vi "load control code.vi"(2 "Switch settings":T7, 3 "Control mode":T6 {"6"."Code"."Data average interval" min=0.0 format="%^#_3g"; "6"."PWM"."Fractional Duty" min=0.0 max=1.0; "5"."Code"."Data average interval" min=0.0 format="%^#_3g"; "5"."PWM"."Fractional Duty" min=0.0 max=1.0; "4"."Code"."Data average interval" min=0.0 format="%^#_3g"; "4"."PWM"."Fractional Duty" min=0.0 max=1.0; "3"."Code"."Data average interval" min=0.0 format="%^#_3g"; "3"."PWM"."Fractional Duty" min=0.0 max=1.0; "2"."Code"."Data average interval" min=0.0 format="%^#_3g"; "2"."PWM"."Fractional Duty" min=0.0 max=1.0; "1"."Code"."Data average interval" min=0.0 format="%^#_3g"; "1"."PWM"."Fractional Duty" min=0.0 max=1.0; "Pump"."Code"."Data average interval" min=0.0 format="%^#_3g"; "Pump"."PWM"."Fractional Duty" min=0.0 max=1.0}) -> (0 "code okay":bool[](array[boolean]), 1 "Control mode out":T5 {"[6]"."Code"."Data average interval" min=0.0 format="%^#_3g"; "[6]"."PWM"."Fractional Duty" min=0.0 max=1.0; "[5]"."Code"."Data average interval" min=0.0 format="%^#_3g"; "[5]"."PWM"."Fractional Duty" min=0.0 max=1.0; "[4]"."Code"."Data average interval" min=0.0 format="%^#_3g"; "[4]"."PWM"."Fractional Duty" min=0.0 max=1.0; "[3]"."Code"."Data average interval" min=0.0 format="%^#_3g"; "[3]"."PWM"."Fractional Duty" min=0.0 max=1.0; "[2]"."Code"."Data average interval" min=0.0 format="%^#_3g"; "[2]"."PWM"."Fractional Duty" min=0.0 max=1.0; "[1]"."Code"."Data average interval" min=0.0 format="%^#_3g"; "[1]"."PWM"."Fractional Duty" min=0.0 max=1.0; "[0]"."Code"."Data average interval" min=0.0 format="%^#_3g"; "[0]"."PWM"."Fractional Duty" min=0.0 max=1.0})   [LabVIEW 2010]
uses:
  Switch wtih PWM code.ctl
  Switch settings PWM.ctl
  PWM.ctl
  type specifier for control code.ctl
  Code.ctl
  Data for Controls.ctl
  Switch control modes.ctl
panel:
  in  "type specifier VI Refnum (for type only)":T1
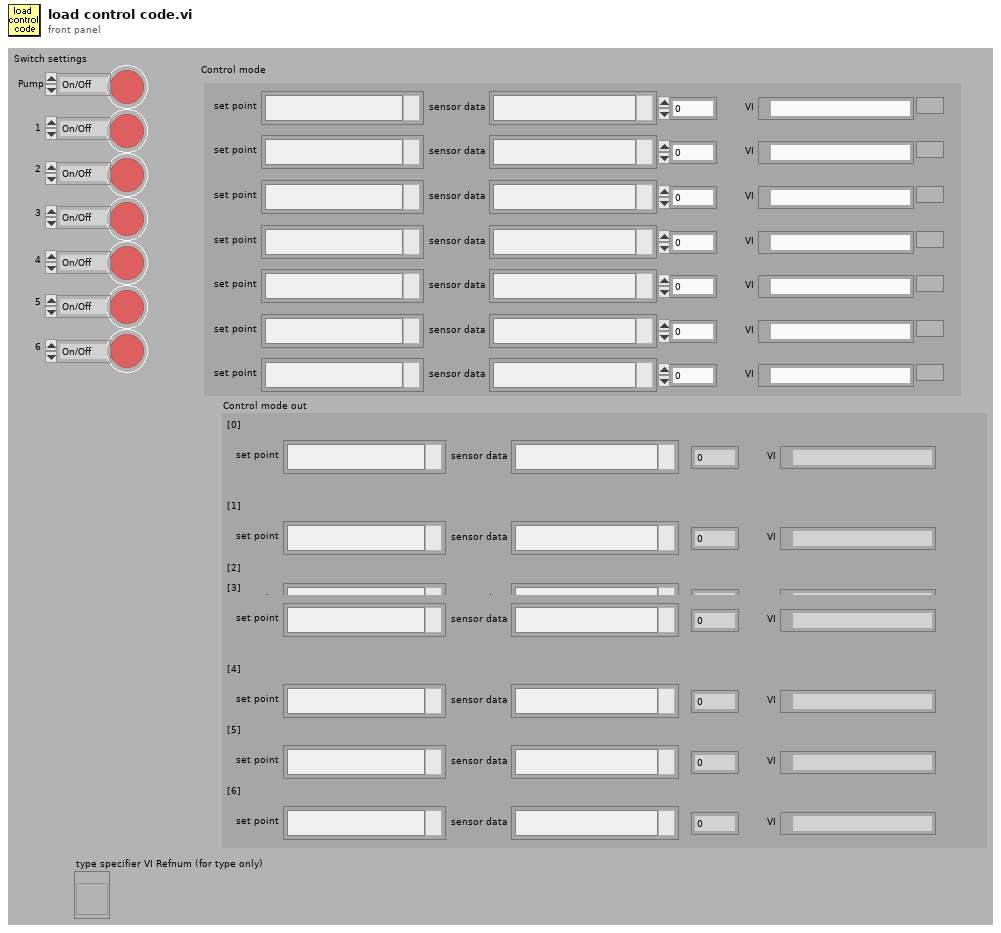
[diagram p1: front panel]
types:
  T1 = typedef "type specifier for control code.ctl" = refnum<vi>
  T2 = typedef "Data for Controls.ctl" = cluster{"PWM":T3, "Code":T4}
  T3 = typedef "PWM.ctl" = cluster{"Fractional Duty":dbl}
  T4 = typedef "Code.ctl" = cluster{"set point":i32[], "VI":path, "sensor data":i32[], "Data average interval":dbl, "code ref":T1}
  T5 = cluster{"[0]":T2, "[1]":T2, "[2]":T2, "[3]":T2, "[4]":T2, "[5]":T2, "[6]":T2}
  T6 = typedef "Switch control modes.ctl" = cluster{"Pump":T2, "1":T2, "2":T2, "3":T2, "4":T2, "5":T2, "6":T2}
  T7 = typedef "Switch settings PWM.ctl" = cluster{"Pump":T8, "1":T8, "2":T8, "3":T8, "4":T8, "5":T8, "6":T8}
  T8 = typedef "Switch wtih PWM code.ctl" = enum16{"On/Off", "Fraction", "Code"}
  T9 = cluster{"Set Point names":string[], "required number of setpoints":u8, "required number of sensors":u8, "Sensor names":string[]}
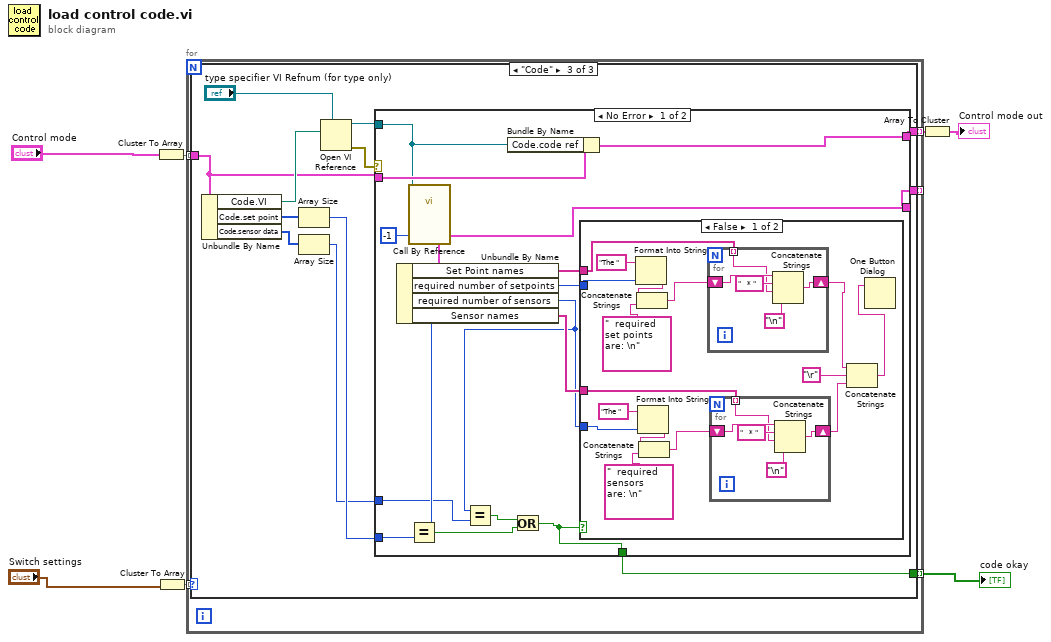
[diagram p0: block diagram]
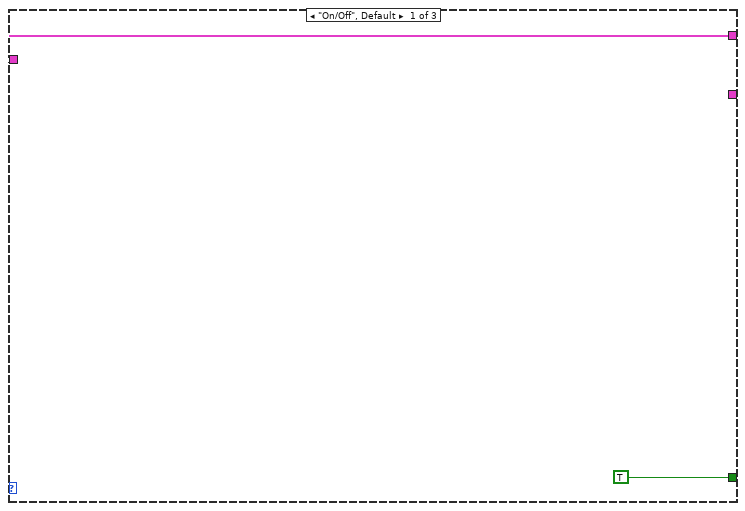
[diagram p2: hidden frame]
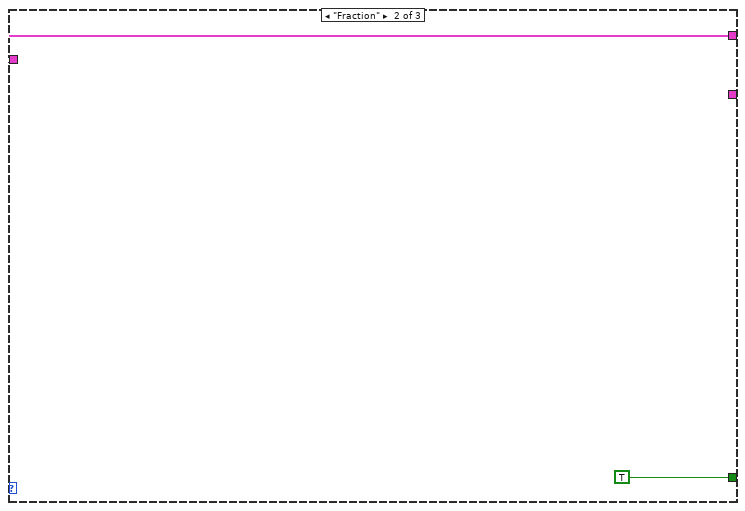
[diagram p3: hidden frame]
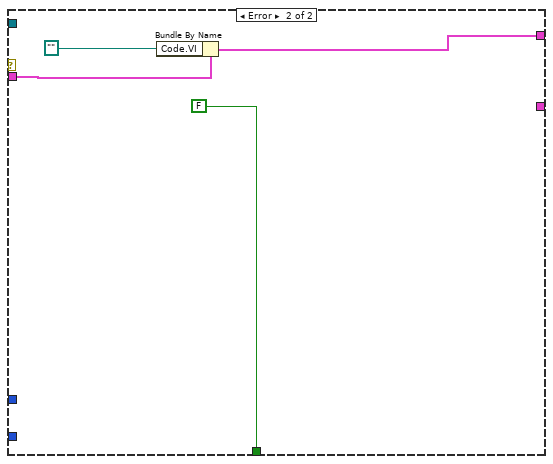
[diagram p5: hidden frame]
diagram:
  n1 = Cluster To Array(cluster="Control mode") -> (array=w7:T2[])
  n2 = Cluster To Array(cluster="Switch settings") -> (array=w6:T8[])
  n3 = for {
    tunnel: w7 -> [w12] mode=indexing
    tunnel: w6 -> [w11] mode=indexing
    tunnel: [w10] -> w5 mode=indexing
    tunnel: [w9] -> w1 mode=indexing
    tunnel: [w8] -> _ mode=indexing
    n4 = case shown="\"Code\"" w11 {
      tunnel: w12 -> [w14 w16 w26]
      tunnel: [w14 w16 w24] -> w10
      tunnel: [TRUE TRUE w23] -> w9
      tunnel: [_ _ w21] -> w8
      frame "On/Off", Default {
      }
      frame "Fraction" {
      }
      frame "Code" {
        n5 = Unbundle By Name(w26) -> ("Code.VI"=w28:path, "Code.set point"=w20:i32[], "Code.sensor data"=w18:i32[])
        n6 = Array Size(array=w20) -> (size(s)=w19:i32)
        n7 = Array Size(array=w18) -> (size(s)=w17:i32)
        n8 = Open VI Reference(type specifier VI Refnum (for type only)="type specifier VI Refnum (for type only)", vi path=w28) -> (vi reference=w25:T1, error out=w27:errorcluster)  [unwired: 4 in]
        n9 = case shown="No Error" w27 {
          tunnel: w26 -> [w42 w72]
          tunnel: w25 -> [w40 _]
          tunnel: [w41 w71] -> w24
          tunnel: [w29 FALSE] -> w23
          tunnel: [w38 _] -> w21
          tunnel: w19 -> [w39 _]
          tunnel: w17 -> [w33 _]
          frame No Error {
            n10 = call-by-ref "?"(reference=w40, "State"=i16 -1) -> ("required data"=w38:T9)  [unwired: 6 in, 3 out]
            n11 = Unbundle By Name(w38) -> ("Set Point names"=w37:string[], "required number of setpoints"=w35:u8, "required number of sensors"=w34:u8, "Sensor names"=w36:string[])
            n12 = Equal?(x=w35, y=w39) -> (x = y?=w31:bool)
            n13 = Equal?(x=w34, y=w33) -> (x = y?=w32:bool)
            n14 = Bundle By Name(cluster=w42, "Code.code ref"=w40) -> (w41:T2)
            n15 = Or(x=w32, y=w31) -> (x .or. y?=w29:bool)
            n16 = case shown="False" w29 {
              tunnel: w35 -> [w55 _]
              tunnel: w37 -> [w53 _]
              tunnel: w36 -> [w44 _]
              tunnel: w34 -> [w43 _]
              frame False {
                n17 = Format Into String(initial string="The ", w55) -> (resulting string=w54:string)  [unwired: 2 in, 1 out]
                n18 = Concatenate Strings(w54, "  required set points are: \n") -> (w56:string)
                n19 = Format Into String(initial string="The ", w43) -> (resulting string=w52:string)  [unwired: 2 in, 1 out]
                n20 = Concatenate Strings(w52, "  required sensors are: \n") -> (w51:string)
                n21 = for {
                  shift-right: [w67] -> w46
                  shift-left: w56 -> [w68]
                  tunnel: w53 -> [w64] mode=indexing
                  n22 = Concatenate Strings(w68, "   * " ("string"), w64, "\n") -> (w67:string)
                }
                n23 = for {
                  shift-right: [w62] -> w47
                  shift-left: w51 -> [w63]
                  tunnel: w44 -> [w59] mode=indexing
                  n24 = Concatenate Strings(w63, "   * " ("string"), w59, "\n") -> (w62:string)
                }
                n25 = Concatenate Strings(w46, "\r", w47) -> (w45:string)
                n26 = One Button Dialog(message=w45) -> ()  [unwired: 1 in, 1 out]
              }
              frame True {
              }
            }
          }
          frame Error {
            n27 = Bundle By Name(cluster=w72, "Code.VI"=path "") -> (w71:T2)
          }
        }
      }
    }
  }
  "code okay" <- w1
  n28 = Array To Cluster(array=w5) -> (cluster=→"Control mode out":T5)
